vi "Write Data to TDMS.vi"(7 "Crash Log (T)":bool, 8 "error in":errorcluster, 9 "Data":T4, 10 "File IO Data In":T1={"System Log File"=path "", "Data File"=path "", "Work Order Folder"=path "", "Runcount File"=path "", "Report Template Folder"=path "", "Report Folder"=path "", "Report File"=path "", "APU Setup Folder"=path "", "Testing State"=FALSE, "Recording State"=FALSE, "APU Select"="<Select>", "Test Information"={"APU Part Number:"="", "Model:"="", "Serial Number:"="", "Customer:"="", "Work Order:"="", "Repair Level:"="", "Pre or Post SB"=""}, "Crash Log Data"=[], "Group Name"="", "APU Setup File"={"Sensor Info"=[], "CMM Table 106"=[], "CMM Table 106B "=[], "Accel Config"=[], "Report Sheet 1"=[], "Report Sheet 2"=[], "Report Sheet 3"=[]}, "APURunCount"=0, "ChannelTagsToLog"=[]}, 11 "Save Data File Ref In":refnum<k34>) -> (0 "error out":errorcluster, 2 "File IO Data Out":T1={"System Log File"=path "", "Data File"=path "", "Work Order Folder"=path "", "Runcount File"=path "", "Report Template Folder"=path "", "Report Folder"=path "", "Report File"=path "", "APU Setup Folder"=path "", "Testing State"=FALSE, "Recording State"=FALSE, "APU Select"="<Select>", "Test Information"={"APU Part Number:"="", "Model:"="", "Serial Number:"="", "Customer:"="", "Work Order:"="", "Repair Level:"="", "Pre or Post SB"=""}, "Crash Log Data"=[], "Group Name"="", "APU Setup File"={"Sensor Info"=[], "CMM Table 106"=[], "CMM Table 106B "=[], "Accel Config"=[], "Report Sheet 1"=[], "Report Sheet 2"=[], "Report Sheet 3"=[]}, "APURunCount"=0, "ChannelTagsToLog"=[]}, 3 "Save Data File Ref Out":refnum<k34>)   [LabVIEW 2018]
doc: "Formats the TMDS file according to the testing type and APU info."
uses:
  Top Level/Shared Controls/Acq Data.ctl
  Top Level/Shared Controls/All Data Cluster.ctl
  Top Level/Shared Controls/Analyzed Data Sets.ctl
  Controller (Host)/Public Controls/Test Information.ctl
  Controller (Host)/Controller (Host).lvlib
  Controller (Host)/Public Controls/APU Select.ctl
  Private Controls/File IO Data.ctl
  File IO.lvlib
  Top Level/Shared Controls/APU Setup File.ctl
panel:
  # "Test Information:"
  # "Test Information:"
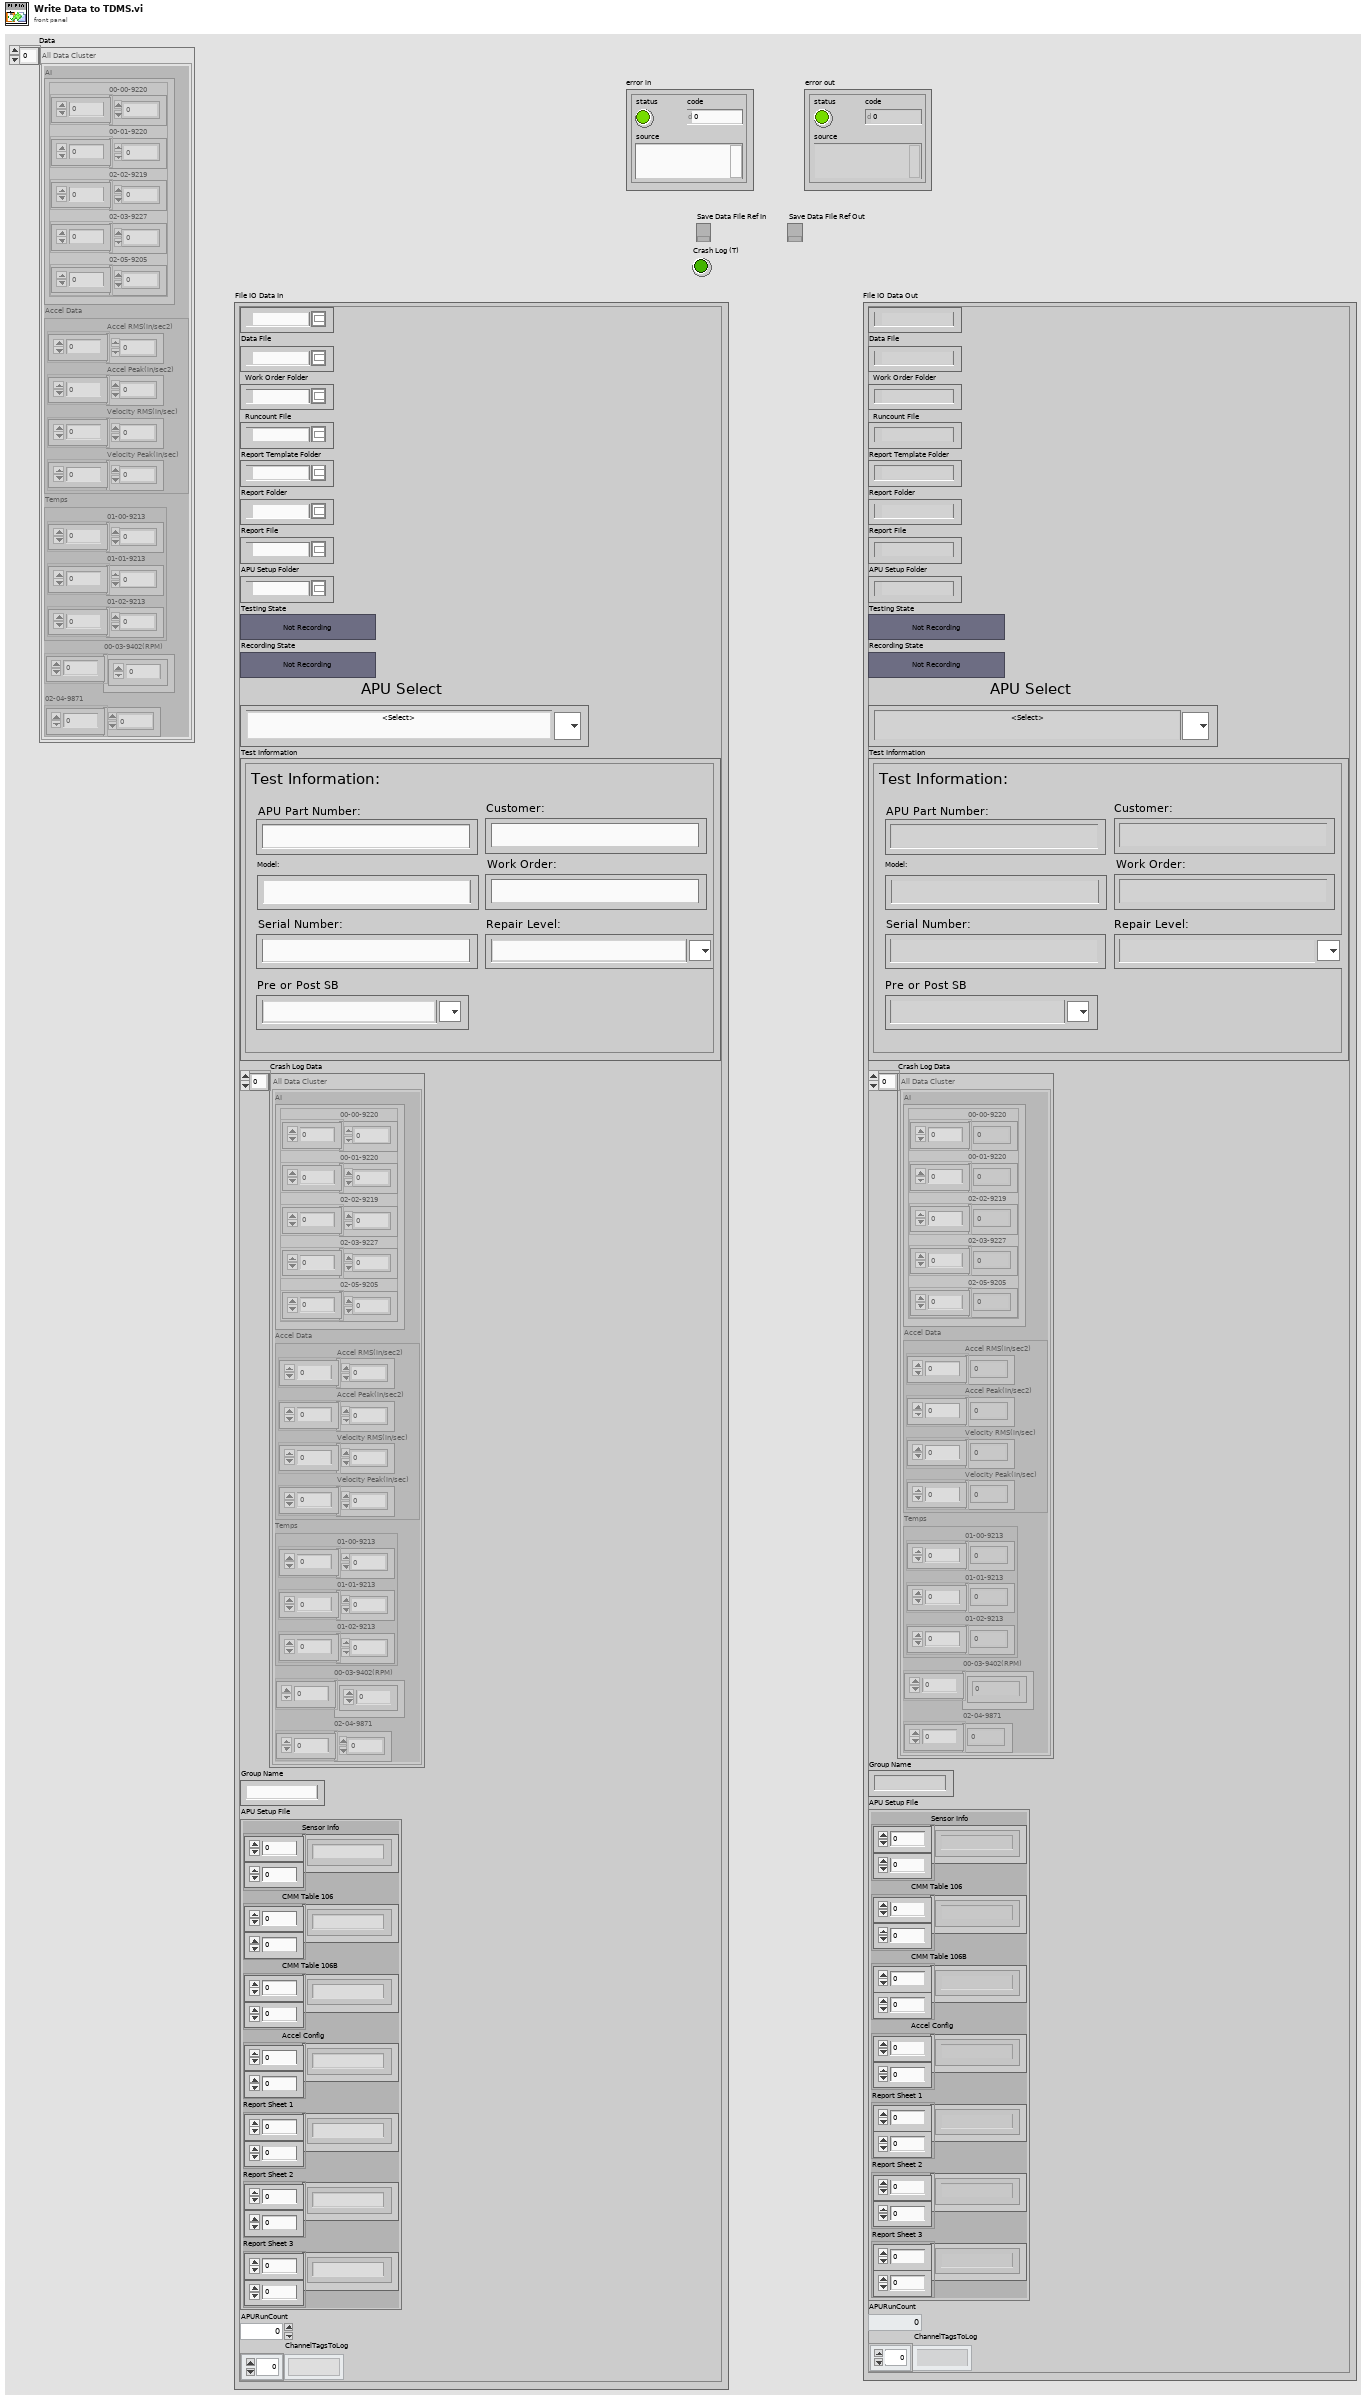
[diagram p1: front panel]
types:
  T1 = typedef "File IO.lvlib/File IO Data.ctl" = cluster{"System Log File":path, "Data File":path, "Work Order Folder":path, "Runcount File":path, "Report Template Folder":path, "Report Folder":path, "Report File":path, "APU Setup Folder":path, "Testing State":bool, "Recording State":bool, "APU Select":T2, "Test Information":T3, "Crash Log Data":T4, "Group Name":string, "APU Setup File":T7, "APURunCount":u32, "ChannelTagsToLog":string[]}
  T2 = typedef "Controller (Host).lvlib/APU Select.ctl" = string
  T3 = typedef "Controller (Host).lvlib/Test Information.ctl" = cluster{"APU Part Number:":string, "Model:":string, "Serial Number:":string, "Customer:":string, "Work Order:":string, "Repair Level:":string, "Pre or Post SB":string}
  T4 = typedef "Analyzed Data Sets.ctl" = T5[]
  T5 = typedef "All Data Cluster.ctl" = cluster{"AI":T6, "Accel Data":cluster{"Accel RMS(in/sec2)":dbl[], "Accel Peak(in/sec2)":dbl[], "Velocity RMS(in/sec)":dbl[], "Velocity Peak(in/sec)":dbl[]}, "Temps":cluster{"01-00-9213":dbl[], "01-01-9213":dbl[], "01-02-9213":dbl[]}, "00-03-9402(RPM)":dbl[], "02-04-9871":dbl[]}
  T6 = typedef "Acq Data.ctl" = cluster{"00-00-9220":dbl[], "00-01-9220":dbl[], "02-02-9219":dbl[], "02-03-9227":dbl[], "02-05-9205":dbl[]}
  T7 = typedef "APU Setup File.ctl" = cluster{"Sensor Info":string[][], "CMM Table 106":string[][], "CMM Table 106B ":string[][], "Accel Config":string[][], "Report Sheet 1":string[][], "Report Sheet 2":string[][], "Report Sheet 3":string[][]}
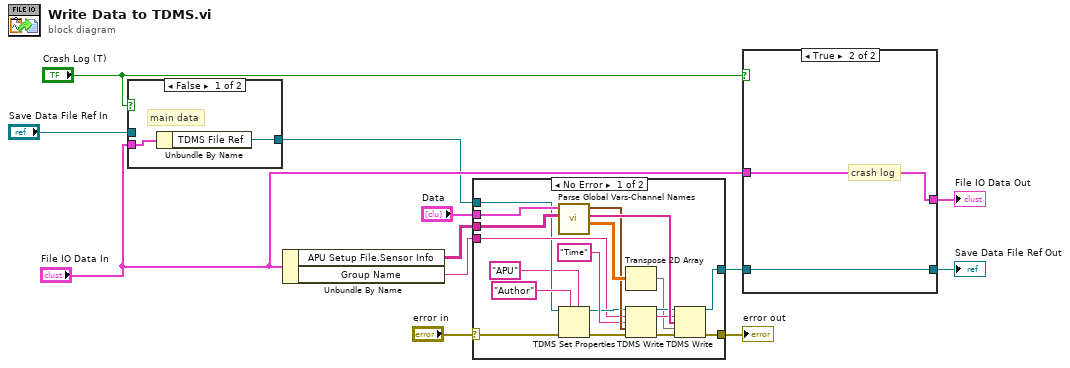
[diagram p0: block diagram]
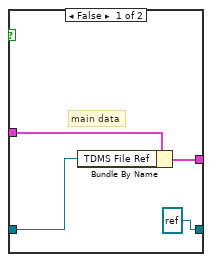
[diagram p3: hidden frame]
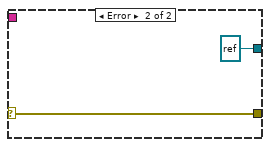
[diagram p4: hidden frame]
diagram:
  n1 = case shown="False" "Crash Log (T)" {
    tunnel: "File IO Data In" -> [w14 _]
    tunnel: [w13 w15] -> w3
    tunnel: "Save Data File Ref In" -> [_ w15]
    frame False {
      # "main data"
      n2 = Unbundle By Name(w14) -> ("TDMS File Ref"=w13:refnum<k34>)
    }
    frame True {
      # "crash log"
    }
  }
  n3 = Unbundle By Name("File IO Data In") -> ("APU Setup File.Sensor Info"=w6:string[][], "Group Name"=w9:string)
  n4 = case shown="No Error" "error in" {
    selector: "error in" -> [w23 w36]
    tunnel: [w33 w36] -> w11
    tunnel: w6 -> [w18 _]
    tunnel: [w34 refnum<k34> refnum ("tdms file out")] -> w7
    tunnel: "Data" -> [w19 _]
    tunnel: w9 -> [w20 _]
    tunnel: w3 -> [w17 _]
    frame No Error {
      n5 = call "Parse Global Vars-Channel Names.vi"("2D Sensor Info"=w18, "Data"=w19) -> ("Data Array"=w28:dbl[][], "Channel Names Array"=w32:string[], "Timestamp Array"=w26:timestamp[])  [unwired: 7 in]
      n6 = TDMS Set Properties(5:"APU", 7:"Author", 8:w23, 11:w17) -> (0:w22:errorcluster, 3:w21:refnum<k34>)  [unwired: 2 in, 2 out]
      n7 = Transpose 2D Array(2D array=w28) -> (transposed array=w27:dbl[][])
      n8 = TDMS Write(0:w21, 5:w20, 7:"Time", 9:w26, 11:w22) -> (4:w31:refnum<k34>, 6:w29:string, 15:w30:errorcluster)  [unwired: 1 in, 1 out]
      n9 = TDMS Write(0:w31, 5:w29, 7:w32, 9:w27, 11:w30) -> (4:w34:refnum<k34>, 15:w33:errorcluster)  [unwired: 1 in, 2 out]
    }
    frame Error {
    }
  }
  "error out" <- w11
  n10 = case shown="True" "Crash Log (T)" {
    tunnel: "File IO Data In" -> [w40 w42]
    tunnel: [w39 w42] -> w8
    tunnel: w7 -> [w38 w41]
    tunnel: [refnum<k34> refnum ("tdms file out") w41] -> w5
    frame False {
      # "main data"
      n11 = Bundle By Name(cluster=w40, "TDMS File Ref"=w38) -> (w39:T1)
    }
    frame True {
      # "crash log"
    }
  }
  "File IO Data Out" <- w8
  "Save Data File Ref Out" <- w5
